vi "总磷数据时间处理.vi"(9 "总磷修正数据输入":T1 {"单位" items=["ug/L", "mg/L", "ppm", "mg/m3", "cm", "ppb", "ug/m3", "%", "nmol/mol", "umol/mol", "MPN/L", "MPN/100ml", "ng/m3", "NTU", "无量纲", "ms/cm", "us/cm", "℃", "mV", "万个/L"]}, 10 "总氮原始数据":T1 {"单位" items=["ug/L", "mg/L", "ppm", "mg/m3", "cm", "ppb", "ug/m3", "%", "nmol/mol", "umol/mol", "MPN/L", "MPN/100ml", "ng/m3", "NTU", "无量纲", "ms/cm", "us/cm", "℃", "mV", "万个/L"]}, 11 "总磷原始数据":T1 {"单位" items=["ug/L", "mg/L", "ppm", "mg/m3", "cm", "ppb", "ug/m3", "%", "nmol/mol", "umol/mol", "MPN/L", "MPN/100ml", "ng/m3", "NTU", "无量纲", "ms/cm", "us/cm", "℃", "mV", "万个/L"]}) -> (3 "总磷修正数据输出":T1 {"单位" items=["ug/L", "mg/L", "ppm", "mg/m3", "cm", "ppb", "ug/m3", "%", "nmol/mol", "umol/mol", "MPN/L", "MPN/100ml", "ng/m3", "NTU", "无量纲", "ms/cm", "us/cm", "℃", "mV", "万个/L"]})   [LabVIEW 2016, in "斯坦道总磷总氮.lvlib"]
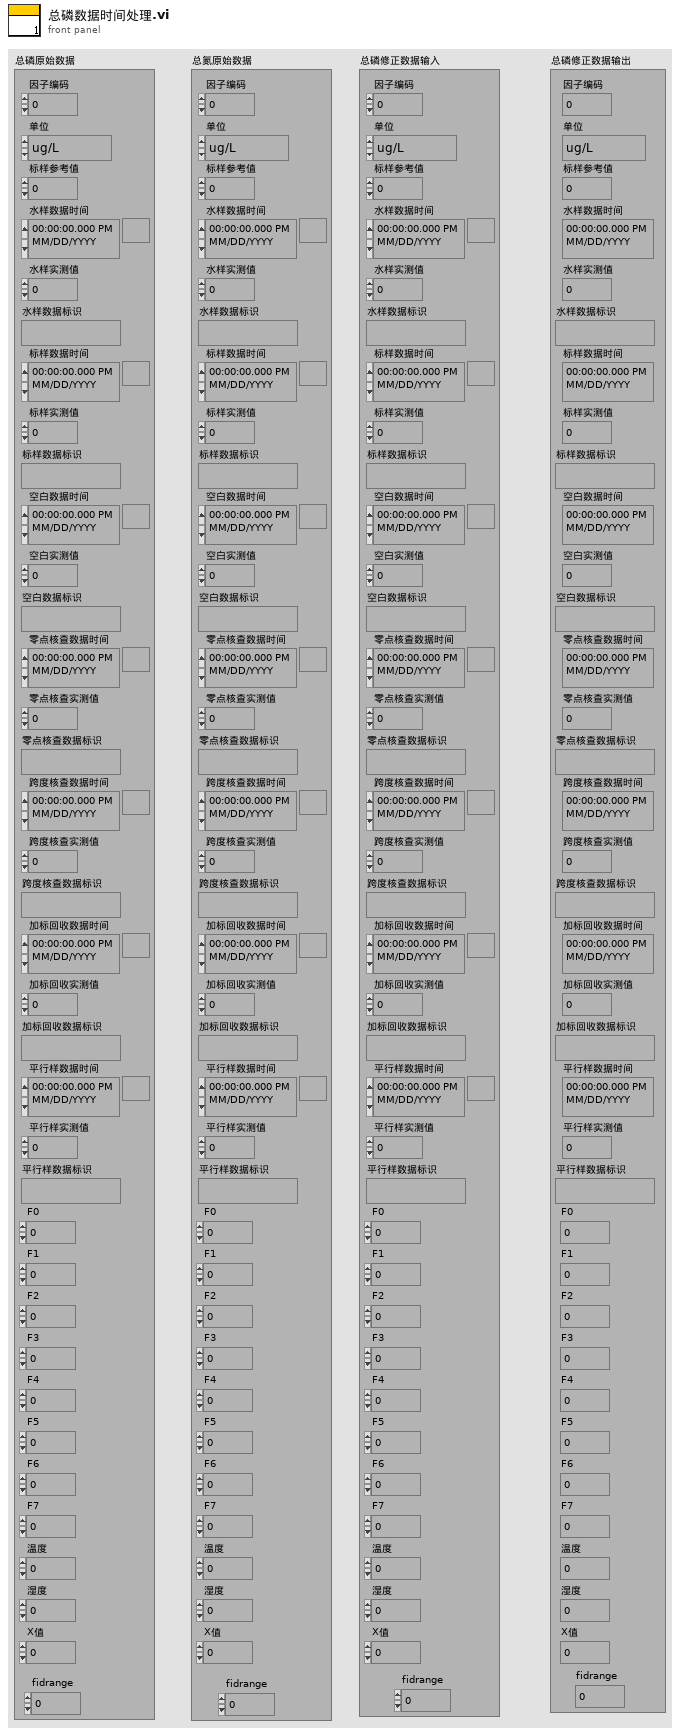
[diagram p1: front panel]
types:
  T1 = cluster{"因子编码":u32, "单位":u16, "标样参考值":sgl, "水样数据时间":timestamp, "水样实测值":sgl, "水样数据标识":string, "标样数据时间":timestamp, "标样实测值":sgl, "标样数据标识":string, "空白数据时间":timestamp, "空白实测值":sgl, "空白数据标识":string, "零点核查数据时间":timestamp, "零点核查实测值":sgl, "零点核查数据标识":string, "跨度核查数据时间":timestamp, "跨度核查实测值":sgl, "跨度核查数据标识":string, "加标回收数据时间":timestamp, "加标回收实测值":sgl, "加标回收数据标识":string, "平行样数据时间":timestamp, "平行样实测值":sgl, "平行样数据标识":string, "F0":sgl, "F1":sgl, "F2":sgl, "F3":sgl, "F4":sgl, "F5":sgl, "F6":sgl, "F7":sgl, "温度":sgl, "湿度":sgl, "X值":sgl, "fidrange":u16}
  T2 = cluster{"因子编码":bool, "单位":bool, "标样参考值":bool, "水样数据时间":bool, "水样实测值":bool, "水样数据标识":bool, "标样数据时间":bool, "标样实测值":bool, "标样数据标识":bool, "空白数据时间":bool, "空白实测值":bool, "空白数据标识":bool, "零点核查数据时间":bool, "零点核查实测值":bool, "零点核查数据标识":bool, "跨度核查数据时间":bool, "跨度核查实测值":bool, "跨度核查数据标识":bool, "加标回收数据时间":bool, "加标回收实测值":bool, "加标回收数据标识":bool, "平行样数据时间":bool, "平行样实测值":bool, "平行样数据标识":bool, "F0":bool, "F1":bool, "F2":bool, "F3":bool, "F4":bool, "F5":bool, "F6":bool, "F7":bool, "温度":bool, "湿度":bool, "X值":bool, "fidrange":bool}
  T3 = cluster{"水样数据时间":timestamp, "标样数据时间":timestamp, "空白数据时间":timestamp, "零点核查数据时间":timestamp, "跨度核查数据时间":timestamp, "加标回收数据时间":timestamp, "平行样数据时间":timestamp}
  T4 = cluster{"水样数据时间":dbl, "标样数据时间":dbl, "空白数据时间":dbl, "零点核查数据时间":dbl, "跨度核查数据时间":dbl, "加标回收数据时间":dbl, "平行样数据时间":dbl}
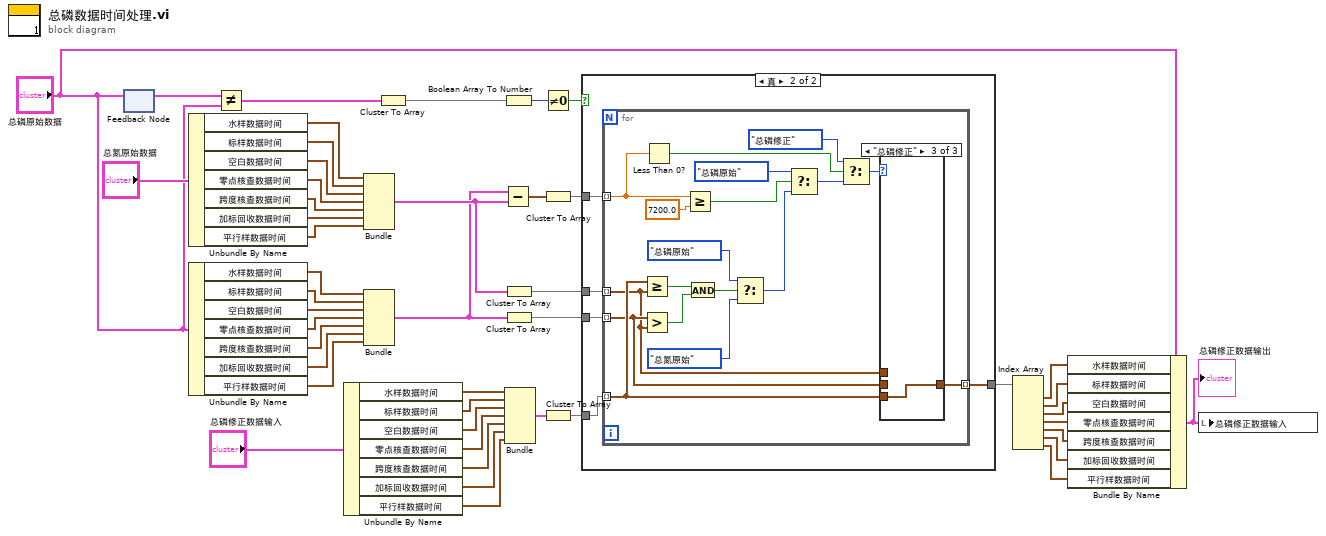
[diagram p0: block diagram]
diagram:
  n1 = feedback-in #1("总磷原始数据") -> ()
  n2 = feedback #1() -> (w7:T1)  [unwired: 1 in]
  n3 = Unbundle By Name("总氮原始数据") -> ("水样数据时间"=w33:timestamp, "标样数据时间"=w34:timestamp, "空白数据时间"=w35:timestamp, "零点核查数据时间"=w36:timestamp, "跨度核查数据时间"=w37:timestamp, "加标回收数据时间"=w38:timestamp, "平行样数据时间"=w39:timestamp)
  n4 = Unbundle By Name("总磷原始数据") -> ("水样数据时间"=w46:timestamp, "标样数据时间"=w45:timestamp, "空白数据时间"=w44:timestamp, "零点核查数据时间"=w43:timestamp, "跨度核查数据时间"=w42:timestamp, "加标回收数据时间"=w41:timestamp, "平行样数据时间"=w40:timestamp)
  n5 = Not Equal?(x=w7, y="总磷原始数据") -> (x != y?=w5:T2)
  n6 = Unbundle By Name("总磷修正数据输入") -> ("水样数据时间"=w26:timestamp, "标样数据时间"=w25:timestamp, "空白数据时间"=w24:timestamp, "零点核查数据时间"=w23:timestamp, "跨度核查数据时间"=w22:timestamp, "加标回收数据时间"=w21:timestamp, "平行样数据时间"=w20:timestamp)
  n7 = Bundle("水样数据时间"=w33, "标样数据时间"=w34, "空白数据时间"=w35, "零点核查数据时间"=w36, "跨度核查数据时间"=w37, "加标回收数据时间"=w38, "平行样数据时间"=w39) -> (w28:T3)  [unwired: 1 in]
  n8 = Bundle("水样数据时间"=w46, "标样数据时间"=w45, "空白数据时间"=w44, "零点核查数据时间"=w43, "跨度核查数据时间"=w42, "加标回收数据时间"=w41, "平行样数据时间"=w40) -> (w8:T3)  [unwired: 1 in]
  n9 = Cluster To Array(cluster=w5) -> (array=w4:bool[])
  n10 = Subtract(x=w8, y=w28) -> (x-y=w31:T4)
  n11 = Boolean Array To Number(Boolean array=w4) -> (number=w3:u32)
  n12 = Cluster To Array(cluster=w28) -> (array=w27:timestamp[])
  n13 = Cluster To Array(cluster=w8) -> (array=w29:timestamp[])
  n14 = Bundle("水样数据时间"=w26, "标样数据时间"=w25, "空白数据时间"=w24, "零点核查数据时间"=w23, "跨度核查数据时间"=w22, "加标回收数据时间"=w21, "平行样数据时间"=w20) -> (w18:T3)  [unwired: 1 in]
  n15 = Not Equal To 0?(x=w3) -> (x != 0?=w2:bool)
  n16 = Cluster To Array(cluster=w31) -> (array=w30:dbl[])
  n17 = Cluster To Array(cluster=w18) -> (array=w17:timestamp[])
  n18 = case shown="真" w2 {
    tunnel: w30 -> [_ w52]
    tunnel: w29 -> [_ w51]
    tunnel: w27 -> [_ w50]
    tunnel: w17 -> [w47 w49]
    tunnel: [w47 w48] -> w9
    frame False {
    }
    frame True {
      n19 = for {
        tunnel: w52 -> [w68] mode=indexing
        tunnel: w51 -> [w60] mode=indexing
        tunnel: w50 -> [w59] mode=indexing
        tunnel: w49 -> [w61] mode=indexing
        tunnel: [w62] -> w48 mode=indexing
        n20 = Greater Or Equal?(x=w61, y=w59) -> (x >= y?=w57:bool)
        n21 = Greater?(x=w60, y=w59) -> (0:w58:bool)
        n22 = Less Than 0?(x=w68) -> (x < 0?=w70:bool)
        n23 = Greater Or Equal?(x=w68, y=7200.0) -> (x >= y?=w63:bool)
        n24 = And(x=w57, y=w58) -> (x .and. y?=w56:bool)
        n25 = Select(t=enum16{"总氮原始", "总磷原始", "总磷修正"}."总磷原始" ("枚举"), s=w56, f=enum16{"总氮原始", "总磷原始", "总磷修正"}."总氮原始" ("枚举")) -> (s? t:f=w53:enum16{"总氮原始", "总磷原始", "总磷修正"})
        n26 = Select(t=enum16{"总氮原始", "总磷原始", "总磷修正"}."总磷原始" ("枚举"), s=w63, f=w53) -> (s? t:f=w65:enum16{"总氮原始", "总磷原始", "总磷修正"})
        n27 = Select(t=enum16{"总氮原始", "总磷原始", "总磷修正"}."总磷修正" ("枚举"), s=w70, f=w65) -> (s? t:f=w64:enum16{"总氮原始", "总磷原始", "总磷修正"})
        n28 = case shown="\"总磷修正\"" w64 {
          tunnel: w59 -> [w71 _ _]
          tunnel: [w71 w72 w73] -> w62
          tunnel: w60 -> [_ w72 _]
          tunnel: w61 -> [_ _ w73]
          frame "总氮原始", Default {
          }
          frame "总磷原始" {
          }
          frame "总磷修正" {
          }
        }
      }
    }
  }
  n29 = Index Array(array=w9) -> (element #1=w16:timestamp, element #2=w15:timestamp, element #3=w14:timestamp, element #4=w13:timestamp, element #5=w12:timestamp, element #6=w11:timestamp, element #7=w10:timestamp)  [unwired: 7 in]
  n30 = Bundle By Name(cluster="总磷原始数据", "水样数据时间"=w16, "标样数据时间"=w15, "空白数据时间"=w14, "零点核查数据时间"=w13, "跨度核查数据时间"=w12, "加标回收数据时间"=w11, "平行样数据时间"=w10) -> (w1:T1)
  "总磷修正数据输出" <- w1
  n31 = local write "总磷修正数据输入"(w1) -> ()
